vi "Evento de usuário.vi"(7 "Enum":T2(ring)=enum."fire - Simular onda", 8 "error in (no error)":errorcluster, 11 "Dados":string) -> (0 "error out":errorcluster, 2 "Event Registration Refnum":refnum<event-registration>)   [LabVIEW 2020]
doc: "Gets the plot data or Sets the FGV value with new data. used to pass data to the HTTP Method"
panel:
  in  "Eventos":T1
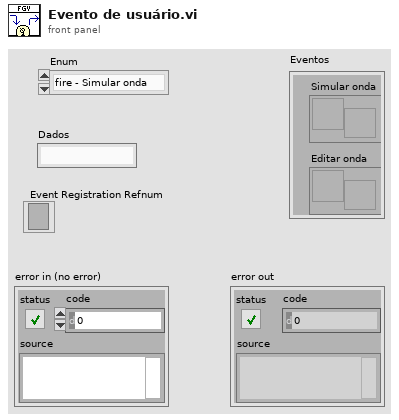
[diagram p1: front panel]
types:
  T1 = cluster{"Simular onda":refnum<user-event>, "Editar onda":refnum<user-event>}
  T2 = enum16{"create", "fire - Simular onda", "fire - Editar onda", "destroy"}
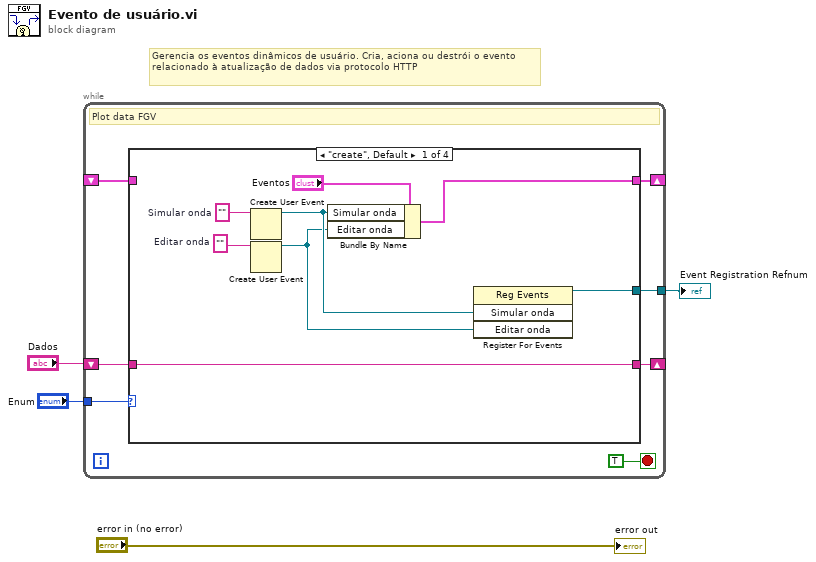
[diagram p0: block diagram]
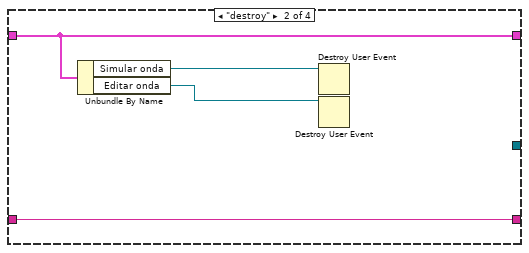
[diagram p2: hidden frame]
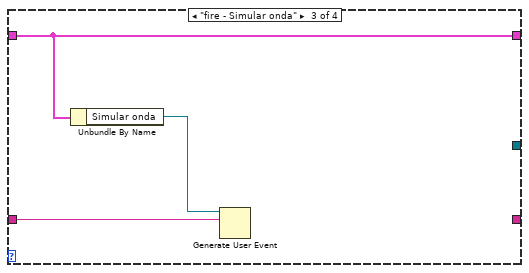
[diagram p3: hidden frame]
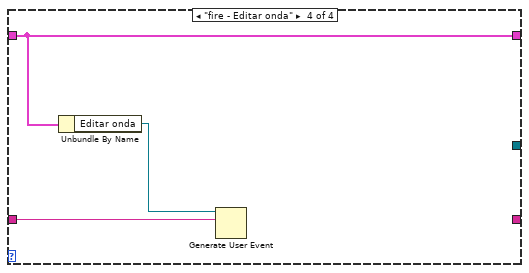
[diagram p4: hidden frame]
diagram:
  # "Gerencia os eventos dinâmicos de usuário. Cria, aciona ou destrói o evento relacionado à atualização de dados via protocolo HTTP"
  n1 = while {
    tunnel: "Enum" -> [w11]
    shift-right: [w9] -> _
    shift-left: _ -> [w8]
    shift-right: [w6] -> _
    shift-left: "Dados" -> [w7]
    tunnel: [w5] -> w1
    stop <- TRUE stop-if-true
    # "Plot data FGV"
    n2 = case shown="\"create\", Default" w11 {
      tunnel: [w15 w23 w24 w29] -> w9
      tunnel: w8 -> [_ w23 w24 w29]
      tunnel: w7 -> [w16 w20 w25 w28]
      tunnel: [w16 w20 _ _] -> w6
      tunnel: [w14 _ _ _] -> w5
      frame "create", Default {
        w18 = ""  # Editar onda
        w19 = ""  # Simular onda
        n3 = Create User Event(user event datatype=w19) -> (user event=w13:refnum<user-event>)  [unwired: 1 in, 1 out]
        n4 = Create User Event(user event datatype=w18) -> (user event=w12:refnum<user-event>)  [unwired: 1 in, 1 out]
        n5 = Bundle By Name(cluster="Eventos", "Simular onda"=w13, "Editar onda"=w12) -> (w15:T1)
        n6 = register-events(w13, w12) -> (reference out=w14:refnum<event-registration>)  [unwired: 2 in, 1 out]
      }
      frame "destroy" {
        n7 = Unbundle By Name(w23) -> ("Simular onda"=w22:refnum<user-event>, "Editar onda"=w21:refnum<user-event>)
        n8 = Destroy User Event(user event=w22) -> ()  [unwired: 1 in, 1 out]
        n9 = Destroy User Event(user event=w21) -> ()  [unwired: 1 in, 1 out]
      }
      frame "fire - Simular onda" {
        n10 = Unbundle By Name(w24) -> ("Simular onda"=w26:refnum<user-event>)
        n11 = Generate User Event(user event=w26, event data cluster=w25) -> ()  [unwired: 2 in, 2 out]
      }
      frame "fire - Editar onda" {
        n12 = Unbundle By Name(w29) -> ("Editar onda"=w27:refnum<user-event>)
        n13 = Generate User Event(user event=w27, event data cluster=w28) -> ()  [unwired: 2 in, 2 out]
      }
    }
  }
  "Event Registration Refnum" <- w1
  "error out" <- "error in (no error)"
